vi "Initialize_Diagonal.vi"(11 "Eigen Value":dbl[](array[numeric])) -> (3 "output matrix":T1)   [LabVIEW 2014]
uses:
  <vilib>/Analysis/Matrix/Datatypes/RealMatrix.ctl
  <vilib>/Analysis/Matrix/NI_Matrix.lvlib
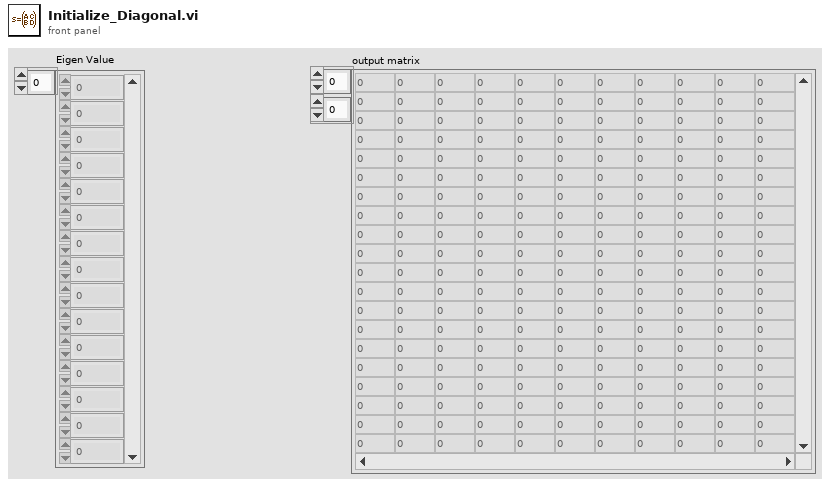
[diagram p1: front panel]
types:
  T1 = typedef "NI_Matrix.lvlib/RealMatrix.ctl" = dbl[][]
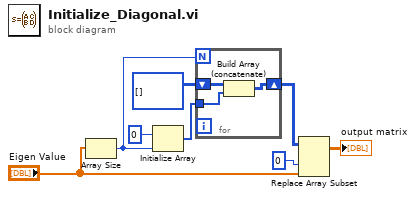
[diagram p0: block diagram]
diagram:
  n1 = Array Size(array="Eigen Value") -> (size(s)=w2:i32)
  n2 = Initialize Array(0 ("dimension size"), w2) -> (w8:i32[])
  n3 = for {
    N: w2 -> [_]
    tunnel: w8 -> [w11]
    shift-right: [w10] -> w6
    shift-left: i32[][] [] -> [w9]
    n4 = Build Array (concatenate)(w9, w11) -> (w10:i32[][])
  }
  n5 = Replace Array Subset(array=w6, new element="Eigen Value", index (col)=0) -> (→"output matrix":T1)  [unwired: 1 in]
